vi "init.vi"(8 "error in (no error)":errorcluster, 9 "SerialNumber":string, 10 "LogPath":path, 11 "CSVTestLog in":refnum<class "CSVTestLog.lvclass">) -> (0 "error out":errorcluster, 3 "CSVTestLog out":refnum<class "CSVTestLog.lvclass">)   [LabVIEW 2015, in "CSVTestLog.lvclass"]
uses:
  CSVTestLog.lvclass
  CSVTestLog.lvclass/CSVTestLog.ctl
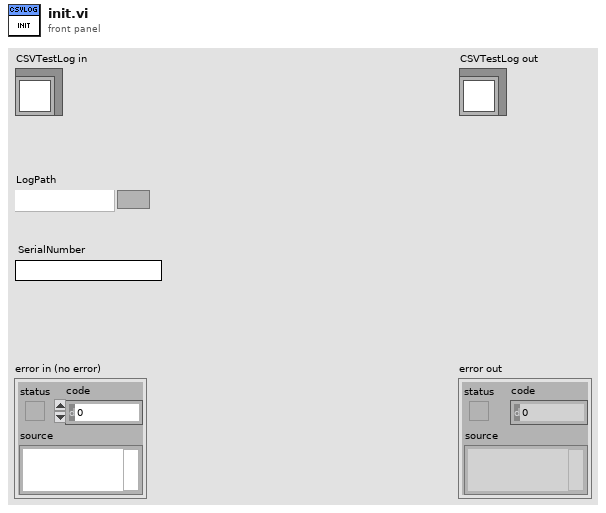
[diagram p1: front panel]
types:
  T1 = enum16{"open", "replace", "create", "open or create", "replace or create", "replace or create with confirmation"}
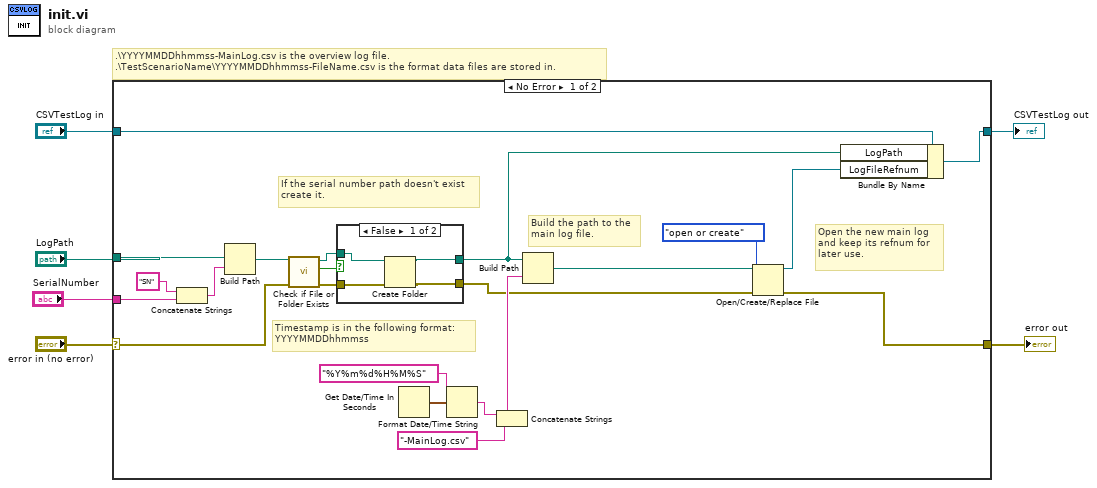
[diagram p0: block diagram]
diagram:
  # ".\\YYYYMMDDhhmmss-MainLog.csv is the overview log file.\n.\\TestScenarioName\\YYYYMMDDhhmmss-FileName.csv is the format data files are stored in."
  n1 = case shown="No Error" "error in (no error)" {
    selector: "error in (no error)" -> [w12 w36]
    tunnel: [w14 w36] -> w5
    tunnel: [w27 w35] -> w3
    tunnel: "CSVTestLog in" -> [w28 w35]
    tunnel: "LogPath" -> [w24 _]
    tunnel: "SerialNumber" -> [w25 _]
    frame No Error {
      # "Build the path to the\nmain log file."
      # "Open the new main log\nand keep its refnum for\nlater use."
      # "Timestamp is in the following format:\nYYYYMMDDhhmmss"
      # "If the serial number path doesn't exist\ncreate it."
      n2 = Concatenate Strings("SN" ("string"), w25) -> (w16:string)
      n3 = Build Path(base path=w24, name or relative path=w16) -> (appended path=w13:path)
      n4 = call <vilib>:"Check if File or Folder Exists.vi"("error in (no error)"=w12, "path"=w13) -> ("error out"=w9:errorcluster, "file or folder exists?"=w11:bool, "dup path"=w10:path)  [unwired: 7 in]
      n5 = case shown="False" w11 {
        tunnel: w10 -> [w32 w34]
        tunnel: w9 -> [w31 w33]
        tunnel: [w30 w33] -> w8
        tunnel: [w29 w34] -> w7
        frame False {
          n6 = Create Folder(path (use dialog)=w32, error in=w31) -> (created path=w29:path, error out=w30:errorcluster)  [unwired: 1 in, 1 out]
        }
        frame True {
        }
      }
      n7 = Get Date/Time In Seconds() -> (seconds since 1Jan1904=w20:timestamp)
      n8 = Format Date/Time String(time format string (%c)="%Y%m%d%H%M%S", seconds (now)=w20) -> (date/time string=w18:string)  [unwired: 1 in]
      n9 = Concatenate Strings(w18, "-MainLog.csv" ("string")) -> (w22:string)
      n10 = Build Path(base path=w7, name or relative path=w22) -> (appended path=w17:path)
      n11 = Open/Create/Replace File(file path (use dialog)=w17, error in=w8, operation (0:open)=T1."open or create") -> (refnum out=w15:refnum<file>, error out=w14:errorcluster)  [unwired: 3 in, 1 out]
      n12 = Bundle By Name(cluster=w28, "LogPath"=w7, "LogFileRefnum"=w15) -> (w27:refnum<class "CSVTestLog.lvclass">)
    }
    frame Error {
    }
  }
  "error out" <- w5
  "CSVTestLog out" <- w3
